vi "Proceed.vi"(7 "component is ready (Y)":bool=TRUE, 8 "error in (no error)":errorcluster, 10 "ProceedMessage":refnum<class "ProceedMessage.lvclass">, 11 "Tomo in":refnum<class "Tomo.lvclass">) -> (0 "error out":errorcluster, 2 "all observers are ready?":bool, 3 "Tomo out":refnum<class "Tomo.lvclass">)   [LabVIEW 2012, in "Tomo.lvclass"]
uses:
  Tomo.lvclass
  <vilib>/Distrio/Murmex/ProceedMessage/ProceedMessage.lvclass
  <vilib>/Distrio/Murmex/StartMessage/StartMessage.lvclass
  <vilib>/Distrio/Murmex/StopMessage/StopMessage.lvclass
  <vilib>/Distrio/Murmex/Murmex/Murmex.lvclass
  <vilib>/Distrio/Murmex/Message/Message.lvclass
panel:
  # "This method is called when the PROCEED\ntrigger is sent. \n\nOverride this method when your component needs to\nrespond to this trigger. \n\nCall parent for proper implementation"
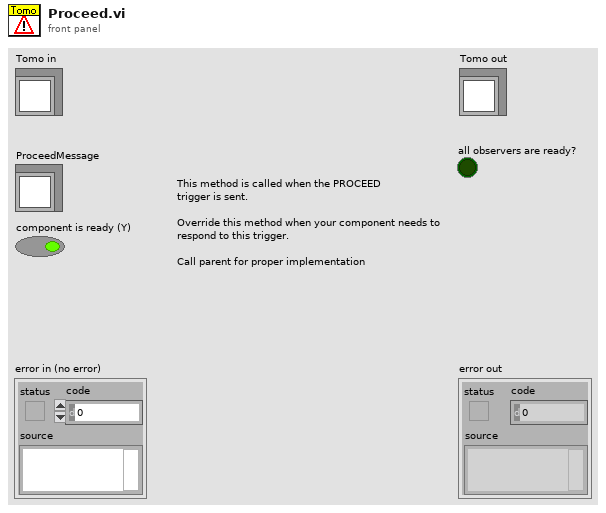
[diagram p1: front panel]
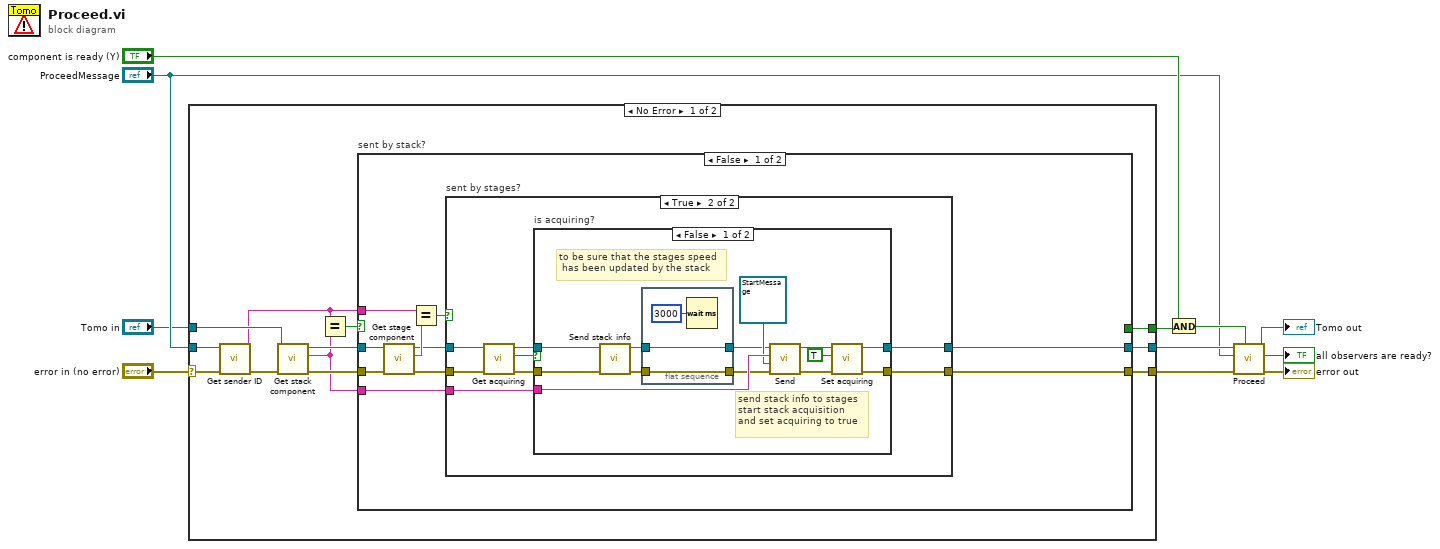
[diagram p0: block diagram]
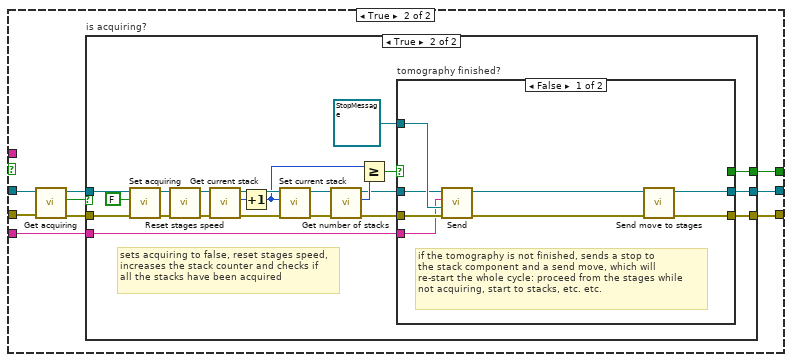
[diagram p4: hidden frame]
diagram:
  n1 = case shown="No Error" "error in (no error)" {
    selector: "error in (no error)" -> [w23 w107]
    tunnel: [w14 w107] -> w10
    tunnel: [w15 w106] -> w9
    tunnel: "ProceedMessage" -> [w22 _]
    tunnel: "Tomo in" -> [w20 w106]
    tunnel: [w12 _] -> w1
    frame No Error {
      n2 = call <vilib>:"Get sender ID.vi"("error in (no error)"=w23, "Message in"=w22) -> ("error out"=w21:errorcluster, "sender"=w18:string)  [unwired: 7 in, 1 out]
      n3 = call-dynamic "Get stack component.vi"("error in (no error)"=w21, "Tomo in"=w20) -> ("error out"=w17:errorcluster, "stack component"=w13:string, "Tomo out"=w16:refnum<class "Tomo.lvclass">)  [unwired: 7 in]
      n4 = Equal?(x=w18, y=w13) -> (x = y?=w19:bool)
      n5 = case "sent by stack?" shown="False" w19 {
        tunnel: w18 -> [w30 _]
        tunnel: w17 -> [w33 w70]
        tunnel: w16 -> [w32 w69]
        tunnel: [w26 w65] -> w15
        tunnel: [w25 w64] -> w14
        tunnel: w13 -> [w24 w63]
        tunnel: [_ w62] -> w12
        frame False {
          n6 = call-dynamic "Get stage component.vi"("error in (no error)"=w33, "Tomo in"=w32) -> ("error out"=w27:errorcluster, "stage component"=w31:string, "Tomo out"=w28:refnum<class "Tomo.lvclass">)  [unwired: 7 in]
          n7 = Equal?(x=w30, y=w31) -> (x = y?=w29:bool)
          n8 = case "sent by stages?" shown="True" w29 {
            tunnel: w28 -> [w35 w42]
            tunnel: w27 -> [w34 w43]
            tunnel: [w35 w38] -> w26
            tunnel: [w34 w37] -> w25
            tunnel: w24 -> [_ w36]
            frame False {
            }
            frame True {
              n9 = call-dynamic "Get acquiring.vi"("error in (no error)"=w43, "Tomo in"=w42) -> ("error out"=w40:errorcluster, "is acquiring?"=w41:bool, "Tomo out"=w39:refnum<class "Tomo.lvclass">)  [unwired: 7 in]
              n10 = case "is acquiring?" shown="False" w41 {
                tunnel: w40 -> [w56 w60]
                tunnel: w39 -> [w48 w61]
                tunnel: [w52 w61] -> w38
                tunnel: [w54 w60] -> w37
                tunnel: w36 -> [w50 _]
                frame False {
                  # "to be sure that the stages speed\n has been updated by the stack"
                  # "send stack info to stages\nstart stack acquisition\nand set acquiring to true"
                  n11 = call-dynamic "Send stack info.vi"("error in (no error)"=w56, "Tomo in"=w48) -> ("error out"=w44:errorcluster, "Tomo out"=w46:refnum<class "Tomo.lvclass">)  [unwired: 8 in]
                  n12 = flat-sequence {
                    tunnel: [w59] -> w47
                    tunnel: w46 -> [w59]
                    tunnel: [w58] -> w45
                    tunnel: w44 -> [w58]
                    frame #0 {
                      n13 = Wait (ms)(milliseconds to wait=u32 3000) -> ()  [unwired: 1 out]
                    }
                  }
                  n14 = call <vilib>:"Send.vi"("error in (no error)"=w45, "Message"=refnum<class "StartMessage.lvclass"> refnum ("Message in"), "recipient"=w50, "Murmex in"=w47) -> ("error out"=w55:errorcluster, "Murmex out"=w53:refnum<class "Tomo.lvclass">)  [unwired: 6 in]
                  n15 = call-dynamic "Set acquiring.vi"("error in (no error)"=w55, "is acquiring?"=TRUE, "Tomo in"=w53) -> ("error out"=w54:errorcluster, "Tomo out"=w52:refnum<class "Tomo.lvclass">)  [unwired: 7 in]
                }
                frame True {
                  # "sent by stages. This proceed \nwill also be relayed by the stack\ncomponent."
                }
              }
            }
          }
        }
        frame True {
          n16 = call-dynamic "Get acquiring.vi"("error in (no error)"=w70, "Tomo in"=w69) -> ("error out"=w66:errorcluster, "is acquiring?"=w68:bool, "Tomo out"=w67:refnum<class "Tomo.lvclass">)  [unwired: 7 in]
          n17 = case "is acquiring?" shown="True" w68 {
            tunnel: w67 -> [w72 w78]
            tunnel: w66 -> [w71 w89]
            tunnel: [w72 w81] -> w65
            tunnel: [w71 w80] -> w64
            tunnel: w63 -> [_ w82]
            tunnel: [_ w76] -> w62
            frame False {
              # "does nothing. This might be a relayed proceed\nwhen the stages have moved to the starting position of \na stack"
            }
            frame True {
              # "sets acquiring to false, reset stages speed,\nincreases the stack counter and checks if\nall the stacks have been acquired"
              n18 = call-dynamic "Set acquiring.vi"("error in (no error)"=w89, "is acquiring?"=FALSE, "Tomo in"=w78) -> ("error out"=w79:errorcluster, "Tomo out"=w74:refnum<class "Tomo.lvclass">)  [unwired: 7 in]
              n19 = call-dynamic "Reset stages speed.vi"("error in (no error)"=w79, "Tomo in"=w74) -> ("error out"=w75:errorcluster, "Tomo out"=w73:refnum<class "Tomo.lvclass">)  [unwired: 8 in]
              n20 = call-dynamic "Get current stack.vi"("error in (no error)"=w75, "Tomo in"=w73) -> ("error out"=w93:errorcluster, "Current stack"=w92:u16, "Tomo out"=w94:refnum<class "Tomo.lvclass">)  [unwired: 7 in]
              n21 = Increment(x=w92) -> (x+1=w87:u16)
              n22 = call-dynamic "Set current stack.vi"("error in (no error)"=w93, "Current stack"=w87, "Tomo in"=w94) -> ("error out"=w91:errorcluster, "Tomo out"=w90:refnum<class "Tomo.lvclass">)  [unwired: 7 in]
              n23 = call-dynamic "Get number of stacks.vi"("error in (no error)"=w91, "Tomo in"=w90) -> ("error out"=w84:errorcluster, "Number of stacks"=w88:u16, "Tomo out"=w85:refnum<class "Tomo.lvclass">)  [unwired: 7 in]
              n24 = Greater Or Equal?(x=w87, y=w88) -> (x >= y?=w86:bool)
              n25 = case "tomography finished?" shown="False" w86 {
                selector: w86 -> [_ w105]
                tunnel: w85 -> [w101 w104]
                tunnel: w84 -> [w100 w103]
                tunnel: refnum<class "StopMessage.lvclass"> refnum ("Message in") -> [w102 _]
                tunnel: w82 -> [w99 _]
                tunnel: [w96 w104] -> w81
                tunnel: [w95 w103] -> w80
                tunnel: [_ w105] -> w76
                frame False {
                  # "if the tomography is not finished, sends a stop to \nthe stack component and a send move, which will \nre-start the whole cycle: proceed from the stages while\nnot acquiring, start to stacks, etc. etc."
                  n26 = call <vilib>:"Send.vi"("error in (no error)"=w100, "Message"=w102, "recipient"=w99, "Murmex in"=w101) -> ("error out"=w97:errorcluster, "Murmex out"=w98:refnum<class "Tomo.lvclass">)  [unwired: 6 in]
                  n27 = call-dynamic "Send move to stages.vi"("error in (no error)"=w97, "Tomo in"=w98) -> ("error out"=w95:errorcluster, "Tomo out"=w96:refnum<class "Tomo.lvclass">)  [unwired: 8 in]
                }
                frame True {
                  # "sets the boolean flag to true,\nallowing the parent method to send\nthe stop to itself and to all the observers"
                }
              }
            }
          }
        }
      }
    }
    frame Error {
    }
  }
  n28 = And(x="component is ready (Y)", y=w1) -> (x .and. y?=w5:bool)
  n29 = call-parent "Proceed.vi"("component is ready (Y)"=w5, "error in (no error)"=w10, "ProceedMessage"="ProceedMessage", "Murmex in"=w9) -> ("error out"=→"error out":errorcluster, "all observers are ready?"=→"all observers are ready?":bool, "Murmex out"=→"Tomo out":refnum<class "Tomo.lvclass">)  [unwired: 5 in]
